vi "CurrentCorrection.vi"(8 "Calib_data":u8[](array[numeric]) format="%02x", 11 "Current_in_mA":u16[](array[numeric])) -> (2 "Correct_Code":u16[](array[numeric]) format="%03x")   [LabVIEW 2016]
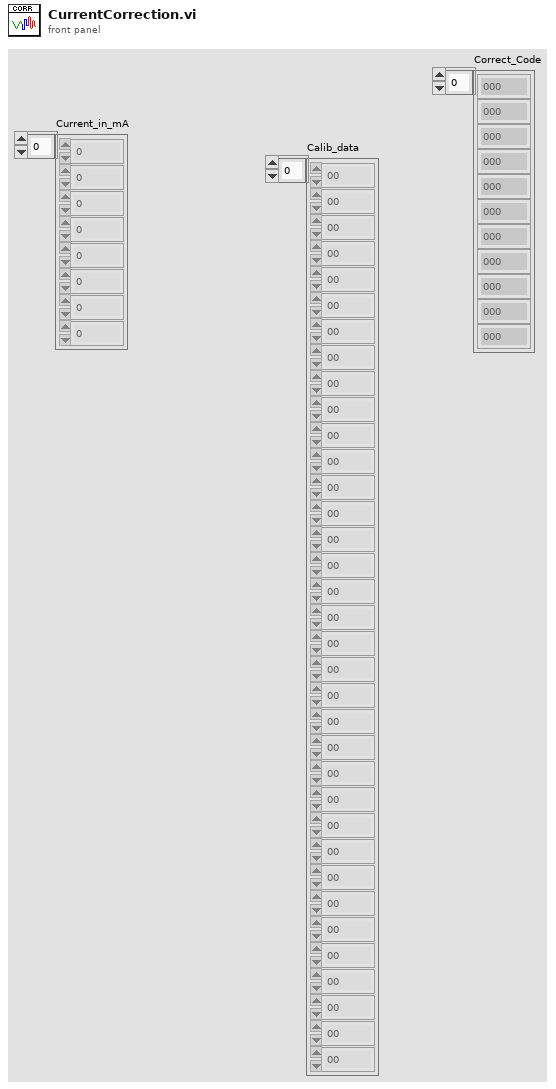
[diagram p1: front panel]
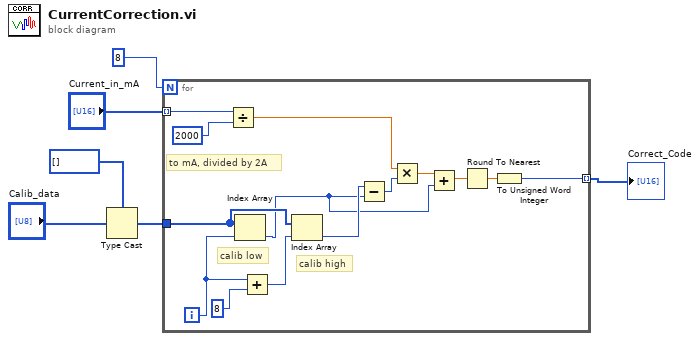
[diagram p0: block diagram]
diagram:
  n1 = Type Cast(type=u16[] [], x="Calib_data") -> (*(type *) &x=w3:u16[])
  n2 = for {
    N: 8 -> [_]
    tunnel: w3 -> [w19]
    tunnel: "Current_in_mA" -> [w15] mode=indexing
    tunnel: [w7] -> w1 mode=indexing
    i -> [w18]
    # "to mA, divided by 2A"
    # "calib high"
    # "calib low"
    n3 = Divide(x=w15, y=u16 2000) -> (x/y=w12:dbl)
    n4 = Index Array(array=w19, index=w18) -> (element=w10:u16)
    n5 = Add(x=w18, y=8) -> (x+y=w17:i32)
    n6 = Index Array(array=w19, index=w17) -> (element=w16:u16)
    n7 = Subtract(x=w16, y=w10) -> (x-y=w13:u16)
    n8 = Multiply(x=w12, y=w13) -> (x*y=w11:dbl)
    n9 = Add(x=w11, y=w10) -> (x+y=w9:dbl)
    n10 = Round To Nearest(number=w9) -> (nearest integer value=w8:dbl)
    n11 = To Unsigned Word Integer(number=w8) -> (unsigned 16bit integer=w7:u16)
  }
  "Correct_Code" <- w1
